vi "Tester receiv.vi"() -> ()   [LabVIEW 2016]
uses:
  <vilib>/Instr/_visa.llb/VISA Configure Serial Port (Instr).vi
panel:
  out "Array":i16[](array[numeric])
  in  "stop":bool
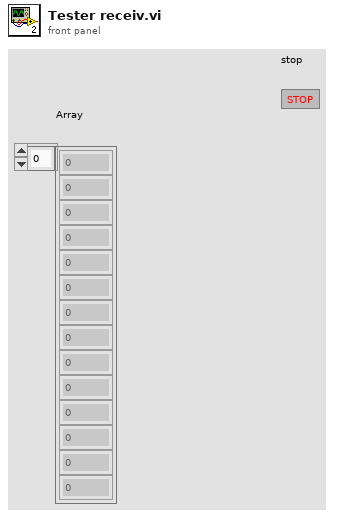
[diagram p1: front panel]
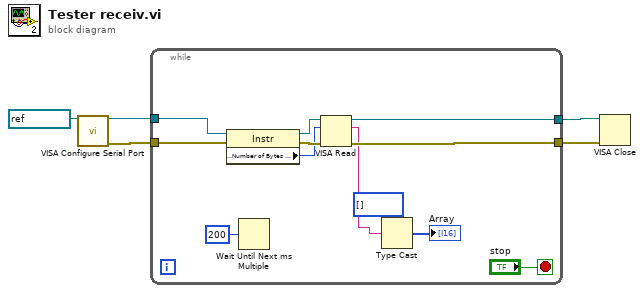
[diagram p0: block diagram]
diagram:
  n1 = call-poly "VISA Configure Serial Port"("VISA resource name"=refnum<visa-resource-name> "COM7") -> ("VISA resource name out"=w5:refnum<visa-resource-name>, "error out"=w4:errorcluster)  [unwired: 13 in]
  n2 = while {
    tunnel: w5 -> [w16]
    tunnel: w4 -> [w15]
    tunnel: [w11] -> w3
    tunnel: [w9] -> w2
    stop <- "stop" stop-if-true
    n3 = property class="Instr"(reference=w16, error in=w15) -> (reference out=w13:refnum<visa-resource-name>, error out=w14:errorcluster, "Serial Settings:Number of Bytes at Serial Port"=w12:u32)
    n4 = Wait Until Next ms Multiple(millisecond multiple=u32 200) -> ()  [unwired: 1 out]
    n5 = VISA Read(VISA resource name=w13, byte count=w12, error in (no error)=w14) -> (VISA resource name out=w9:refnum<visa-resource-name>, read buffer=w6:string, error out=w11:errorcluster)  [unwired: 1 out]
    n6 = Type Cast(type=i16[] [] ("Array"), x=w6) -> (*(type *) &x=→"Array":i16[])
  }
  n7 = VISA Close(VISA resource name=w2, error in (no error)=w3) -> ()  [unwired: 1 out]
